vi "CTI Cryo Read.vi"(8 "error in (no error)":errorcluster, 11 "cRIO I/O Device":refnum<k21>="Mod7\\Port4") -> (0 "error out":errorcluster, 1 "Time since repurge":u8[](array[numeric]), 2 "Cryo On-time":u8[](array[numeric]), 3 "2nd stage temp":u8[](array[numeric]), 4 "Cryo status":u8[](array[numeric]), 5 "1st stage temp":u8[](array[numeric]))   [LabVIEW 2016]
uses:
  <vilib>/rvi/eio/common/nirviEmuTemplateMethod_errors.vi
  <vilib>/eio/EIOMethodNode/EIOMethodNode.xnode
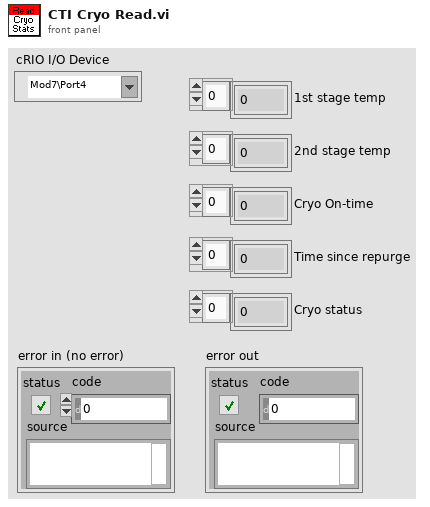
[diagram p1: front panel]
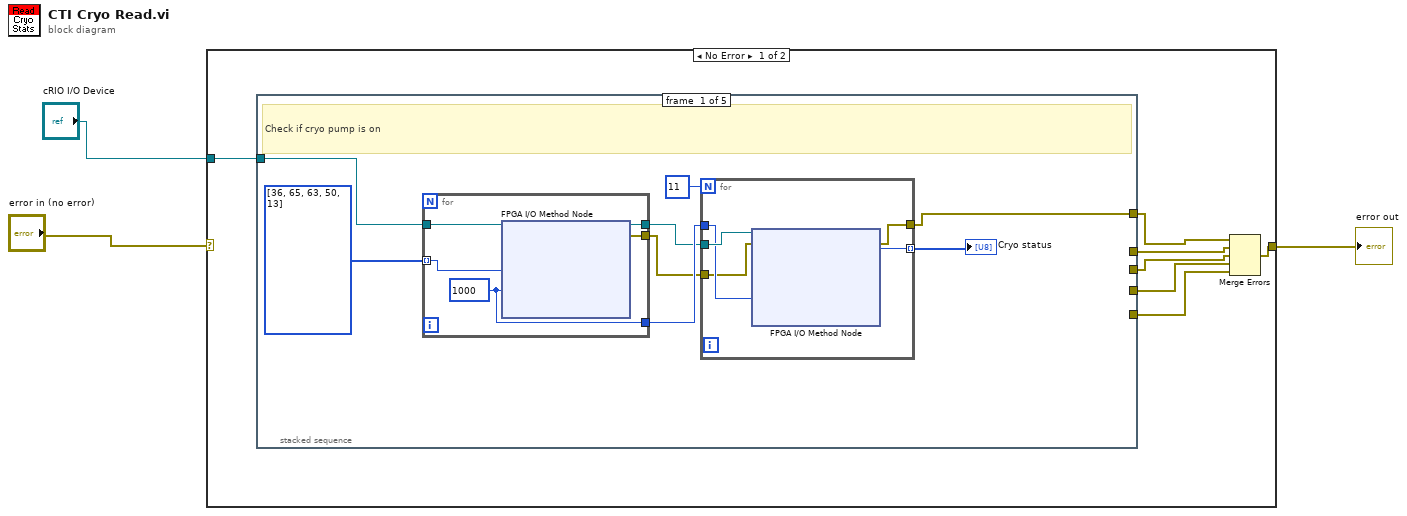
[diagram p0: block diagram]
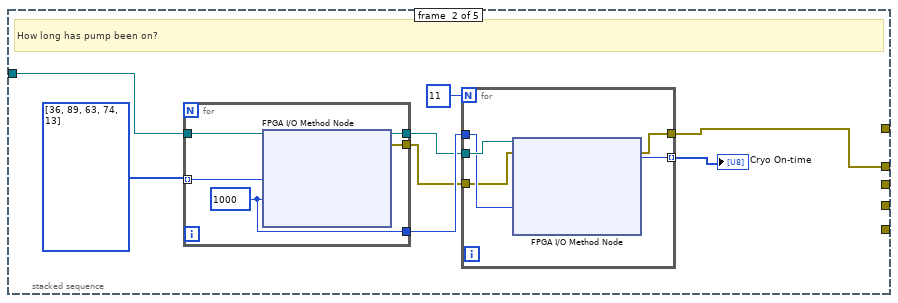
[diagram p2: hidden frame]
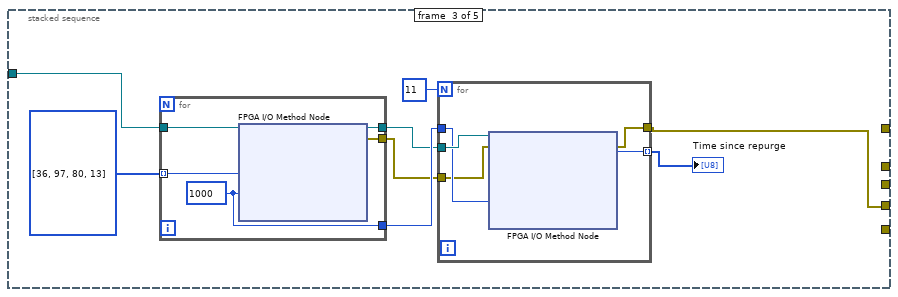
[diagram p3: hidden frame]
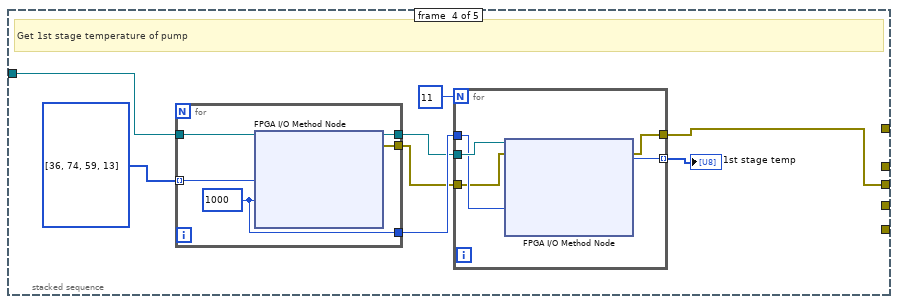
[diagram p4: hidden frame]
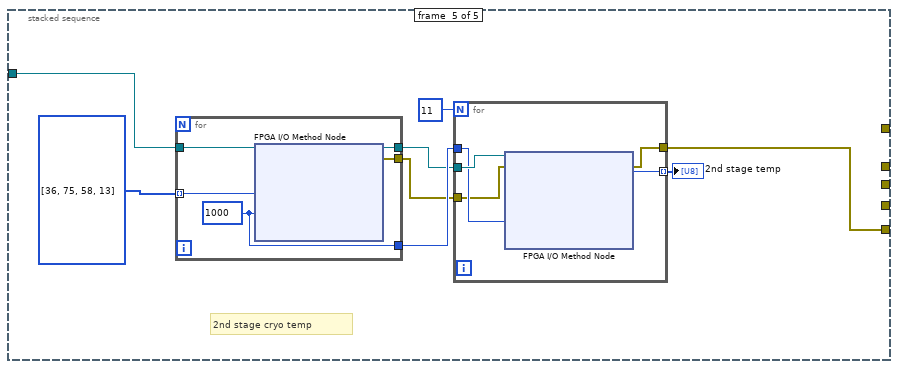
[diagram p5: hidden frame]
diagram:
  n1 = case shown="No Error" "error in (no error)" {
    selector: "error in (no error)" -> [_ w101]
    tunnel: "cRIO I/O Device" -> [w10 _]
    tunnel: [w4 w101] -> w1
    frame No Error {
      n2 = stacked-sequence {
        tunnel: [_ w32 _ _ _] -> w8
        tunnel: [w14 _ _ _ _] -> w9
        tunnel: [_ _ _ w67 _] -> w7
        tunnel: [_ _ w48 _ _] -> w6
        tunnel: [_ _ _ _ w85] -> w5
        tunnel: w10 -> [w12 w30 w50 w65 w84]
        frame #0 {
          # "Check if cryo pump is on"
          n3 = for {
            tunnel: [w26] -> w18
            tunnel: [w28] -> w16
            tunnel: w12 -> [w27]
            tunnel: [w25] -> w15
            tunnel: u8[] [36, 65, 63, 50, 13] ("unsigned byte array") -> [w24] mode=indexing
            w26 = 1000 ("Timeout (ms)")
            n4 = xnode "FPGA I/O Method Node"("FPGA I/O In"=w27, "Data"=w24, "Timeout (ms)"=w26) -> ("error out"=w25:errorcluster, "FPGA I/O Out"=w28:refnum<k21>)  [unwired: 1 in, 1 out]
          }
          n5 = for {
            N: 11 -> [_]
            tunnel: w18 -> [w21]
            tunnel: [w23] -> w13 mode=indexing
            tunnel: w16 -> [w22]
            tunnel: [w19] -> w14
            tunnel: w15 -> [w20]
            n6 = xnode "FPGA I/O Method Node"("error in"=w20, "FPGA I/O In"=w22, "Timeout (ms)"=w21) -> ("error out"=w19:errorcluster, "Data"=w23:u8)  [unwired: 2 out]
          }
          "Cryo status" <- w13
        }
        frame #1 {
          # "How long has pump been on?"
          n7 = for {
            tunnel: [w44] -> w36
            tunnel: u8[] [36, 89, 63, 74, 13] ("unsigned byte array") -> [w43] mode=indexing
            tunnel: [w46] -> w34
            tunnel: w30 -> [w45]
            tunnel: [w42] -> w33
            w44 = 1000 ("Timeout (ms)")
            n8 = xnode "FPGA I/O Method Node"("FPGA I/O In"=w45, "Data"=w43, "Timeout (ms)"=w44) -> ("error out"=w42:errorcluster, "FPGA I/O Out"=w46:refnum<k21>)  [unwired: 1 in, 1 out]
          }
          n9 = for {
            N: 11 -> [_]
            tunnel: w36 -> [w39]
            tunnel: [w41] -> w31 mode=indexing
            tunnel: w34 -> [w40]
            tunnel: [w37] -> w32
            tunnel: w33 -> [w38]
            n10 = xnode "FPGA I/O Method Node"("error in"=w38, "FPGA I/O In"=w40, "Timeout (ms)"=w39) -> ("error out"=w37:errorcluster, "Data"=w41:u8)  [unwired: 2 out]
          }
          "Cryo On-time" <- w31
        }
        frame #2 {
          n11 = for {
            tunnel: [w62] -> w54
            tunnel: u8[] [36, 97, 80, 13] ("unsigned byte array") -> [w61] mode=indexing
            tunnel: [w64] -> w52
            tunnel: w50 -> [w63]
            tunnel: [w60] -> w51
            w62 = 1000 ("Timeout (ms)")
            n12 = xnode "FPGA I/O Method Node"("FPGA I/O In"=w63, "Data"=w61, "Timeout (ms)"=w62) -> ("error out"=w60:errorcluster, "FPGA I/O Out"=w64:refnum<k21>)  [unwired: 1 in, 1 out]
          }
          n13 = for {
            N: 11 -> [_]
            tunnel: w54 -> [w57]
            tunnel: [w59] -> w47 mode=indexing
            tunnel: w52 -> [w58]
            tunnel: [w55] -> w48
            tunnel: w51 -> [w56]
            n14 = xnode "FPGA I/O Method Node"("error in"=w56, "FPGA I/O In"=w58, "Timeout (ms)"=w57) -> ("error out"=w55:errorcluster, "Data"=w59:u8)  [unwired: 2 out]
          }
          "Time since repurge" <- w47
        }
        frame #3 {
          # "Get 1st stage temperature of pump"
          n15 = for {
            tunnel: [w80] -> w72
            tunnel: u8[] [36, 74, 59, 13] ("unsigned byte array") -> [w79] mode=indexing
            tunnel: [w82] -> w70
            tunnel: w65 -> [w81]
            tunnel: [w78] -> w69
            w80 = 1000 ("Timeout (ms)")
            n16 = xnode "FPGA I/O Method Node"("FPGA I/O In"=w81, "Data"=w79, "Timeout (ms)"=w80) -> ("error out"=w78:errorcluster, "FPGA I/O Out"=w82:refnum<k21>)  [unwired: 1 in, 1 out]
          }
          n17 = for {
            N: 11 -> [_]
            tunnel: w72 -> [w75]
            tunnel: [w77] -> w68 mode=indexing
            tunnel: w70 -> [w76]
            tunnel: [w73] -> w67
            tunnel: w69 -> [w74]
            n18 = xnode "FPGA I/O Method Node"("error in"=w74, "FPGA I/O In"=w76, "Timeout (ms)"=w75) -> ("error out"=w73:errorcluster, "Data"=w77:u8)  [unwired: 2 out]
          }
          "1st stage temp" <- w68
        }
        frame #4 {
          # "2nd stage cryo temp"
          n19 = for {
            tunnel: [w98] -> w90
            tunnel: u8[] [36, 75, 58, 13] ("unsigned byte array") -> [w97] mode=indexing
            tunnel: [w100] -> w86
            tunnel: w84 -> [w99]
            tunnel: [w96] -> w83
            w98 = 1000 ("Timeout (ms)")
            n20 = xnode "FPGA I/O Method Node"("FPGA I/O In"=w99, "Data"=w97, "Timeout (ms)"=w98) -> ("error out"=w96:errorcluster, "FPGA I/O Out"=w100:refnum<k21>)  [unwired: 1 in, 1 out]
          }
          n21 = for {
            N: 11 -> [_]
            tunnel: w90 -> [w93]
            tunnel: [w95] -> w87 mode=indexing
            tunnel: w86 -> [w94]
            tunnel: [w91] -> w85
            tunnel: w83 -> [w92]
            n22 = xnode "FPGA I/O Method Node"("error in"=w92, "FPGA I/O In"=w94, "Timeout (ms)"=w93) -> ("error out"=w91:errorcluster, "Data"=w95:u8)  [unwired: 2 out]
          }
          "2nd stage temp" <- w87
        }
      }
      n23 = Merge Errors(w9, w8, w7, w6, w5) -> (w4:errorcluster)
    }
    frame Error {
    }
  }
  "error out" <- w1
